vi "Center Scanner.vi"(7 "Reset":bool, 8 "error in (no error)":errorcluster, 9 "PrevY":u32, 10 "PrevX":u32, 11 "Refnum in":T1) -> (0 "Y":u16, 2 "X":u16, 3 "Refnum out":T1)   [LabVIEW 2015]
uses:
  <vilib>/vision/Image Controls.llb/IMAQ Image.ctl
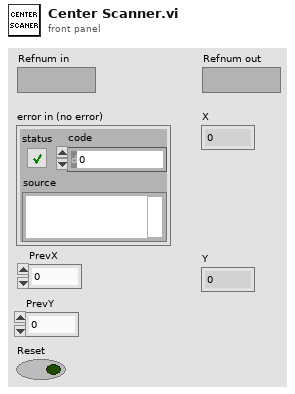
[diagram p1: front panel]
types:
  T1 = typedef "IMAQ Image.ctl" = refnum<image>
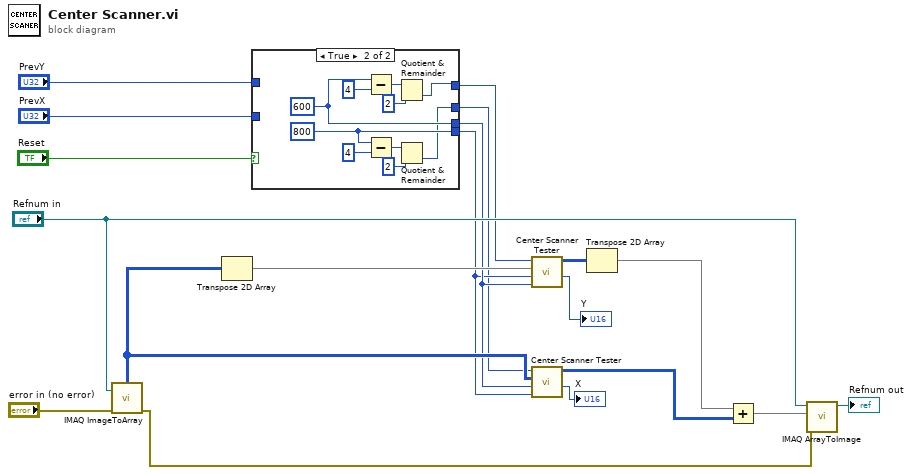
[diagram p0: block diagram]
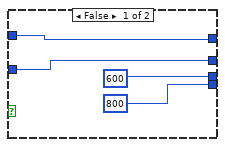
[diagram p2: hidden frame]
diagram:
  n1 = call "IMAQ ImageToArray"("error in (no error)"="error in (no error)", "Image"="Refnum in") -> ("error out"=w16:errorcluster, "Image Pixels (U8)"=w18:u8[][])  [unwired: 2 in, 3 out]
  n2 = Transpose 2D Array(2D array=w18) -> (transposed array=w12:u8[][])
  n3 = case shown="True" "Reset" {
    tunnel: [u16 600 ("Width") w30] -> w8
    tunnel: [w21 w25] -> w7
    tunnel: [u16 800 ("Hight") w26] -> w6
    tunnel: [w20 w24] -> w5
    tunnel: "PrevY" -> [w21 _]
    tunnel: "PrevX" -> [w20 _]
    frame False {
    }
    frame True {
      w26 = u16 800 ("Hight")
      w30 = u16 600 ("Width")
      n4 = Subtract(x=w30, y=u16 4) -> (x-y=w33:u16)
      n5 = Subtract(x=w26, y=u16 4) -> (x-y=w27:u16)
      n6 = Quotient & Remainder(x=w33, y=u32 2) -> (floor(x/y)=w25:u32)  [unwired: 1 out]
      n7 = Quotient & Remainder(x=w27, y=u32 2) -> (floor(x/y)=w24:u32)  [unwired: 1 out]
    }
  }
  n8 = call "Center Scanner Tester.vi"("Hight"=w8, "Width"=w6, "ImageIn"=w12, "StartLine"=w7) -> ("HorCenter"=→"Y":u16, "ImgOut"=w13:u8[][])  [unwired: 6 in]
  n9 = call "Center Scanner Tester.vi"("Hight"=w6, "Width"=w8, "ImageIn"=w18, "StartLine"=w5) -> ("HorCenter"=→"X":u16, "ImgOut"=w11:u8[][])  [unwired: 6 in]
  n10 = Transpose 2D Array(2D array=w13) -> (transposed array=w10:u8[][])
  n11 = Add(x=w10, y=w11) -> (x+y=w1:u8[][])
  n12 = call "IMAQ ArrayToImage"("error in (no error)"=w16, "Image Pixels (U8)"=w1, "Image"="Refnum in") -> ("Image Out"=→"Refnum out":T1)  [unwired: 7 in, 1 out]
